vi "Read Persistent Unified Actor.vi"(11 "Attributes in":refnum<class "Attributes.lvclass">) -> (2 "Persistent Unified Actor":refnum<class "Actor.lvclass">)   [LabVIEW 2025, in "jettl.lvlib" / "Attributes.lvclass"]
uses:
  Attributes.lvclass
  Actor/Actor.lvclass
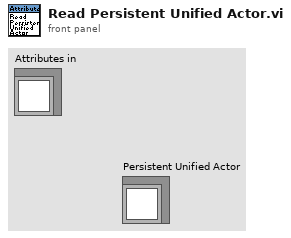
[diagram p1: front panel]
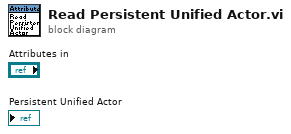
[diagram p0: block diagram]
diagram:
